vi "svc_Copy Array Subset (Index).vi"(8 "error in (no error)":errorcluster, 9 "length (-1 = all)":i32=-1 min=-1 step=1, 10 "start index (0)":i32 step=1, 11 "Y":dbl[](array[numeric])) -> (0 "error out":errorcluster, 1 "actual length":i32, 2 "actual start index":i32, 3 "Y subset":dbl[](array[numeric]), 4 "end reached":bool)   [LabVIEW 2017]
doc: "Returns a portion of the waveform of the <B>start index</B> and <B>length</B> values. When you wire a waveform to this VI, the waveform automatically resizes to display <B>start index</B> inputs for the waveform."
uses:
  <vilib>/addons/_NISVFA/_Shared subVIs/Common/svc_Conditional Merge Error.vi
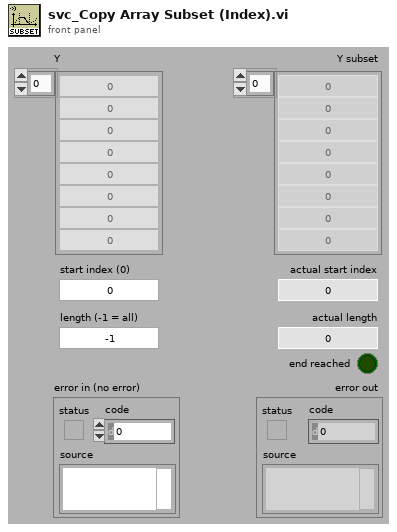
[diagram p1: front panel]
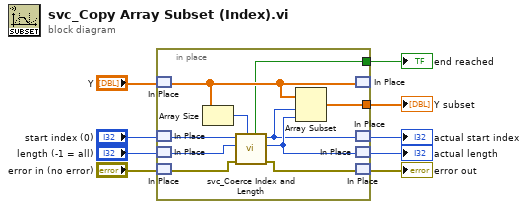
[diagram p0: block diagram]
diagram:
  n1 = in-place {
    in-place-border: [w16] -> w4
    in-place-border: [w19] -> w3
    n2 = in-place-match #1("Y") -> (w18:dbl[])
    n3 = in-place-match #2("start index (0)") -> (w13:i32)
    n4 = in-place-match #3("length (-1 = all)") -> (w15:i32)
    n5 = in-place-match #4("error in (no error)") -> (w12:errorcluster)
    n6 = Array Size(array=w18) -> (size(s)=w17:i32)
    n7 = call <vilib>:"svc_Coerce Index and Length.vi"("input length"=w17, "error in (no error)"=w12, "subset length (-1 = all)"=w15, "subset start index (0)"=w13) -> ("error out"=w11:errorcluster, "actual subset length"=w14:i32, "actual start index"=w10:i32, "end reached"=w16:bool)  [unwired: 4 in]
    n8 = Array Subset(array=w18, index=w10, length=w14) -> (w19:dbl[])
    n9 = in-place-match #1(w18) -> ()  [unwired: 1 out]
    n10 = in-place-match #2(w10) -> (→"actual start index":i32)
    n11 = in-place-match #3(w14) -> (→"actual length":i32)
    n12 = in-place-match #4(w11) -> (→"error out":errorcluster)
  }
  "Y subset" <- w3
  "end reached" <- w4
